vi "Probability.vi"   [LabVIEW 2016]
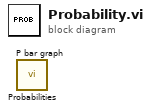
[diagram p0: block diagram]
diagram:
  n1 = call "Probabilities.vi"() -> ()  [unwired: 11 in, 1 out]
  n2 = call "P bar graph.vi"() -> ()  [unwired: 12 in]
